vi "Log_TimePath.vi"(8 "error in (no error)":errorcluster) -> (0 "error out":errorcluster, 3 "result string":string)   [LabVIEW 2013]
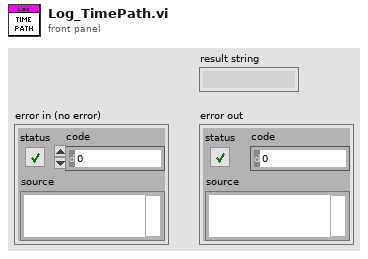
[diagram p1: front panel]
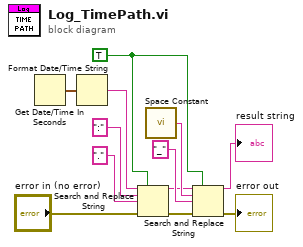
[diagram p0: block diagram]
diagram:
  w8 = TRUE ("replace all? (F)")
  n1 = Get Date/Time In Seconds() -> (seconds since 1Jan1904=w6:timestamp)
  n2 = Format Date/Time String(seconds (now)=w6) -> (date/time string=w2:string)  [unwired: 2 in]
  n3 = Search and Replace String(replace all?=w8, input string=w2, search string=":", replace string="." ("replace string (\"\")"), error in="error in (no error)") -> (result string=w3:string, error out=w7:errorcluster)  [unwired: 3 in, 2 out]
  n4 = call <vilib>:"Space Constant.vi"() -> ("String"=w5:string)
  n5 = Search and Replace String(replace all?=w8, input string=w3, search string=w5, replace string="_" ("replace string (\"\")"), error in=w7) -> (result string=→"result string":string, error out=→"error out":errorcluster)  [unwired: 3 in, 2 out]
